vi "Main On Compile Action VI_Parse RTs.vi"(7 "Autocreate Rx timestamp chans?":bool, 8 "error in":errorcluster, 10 "Channel Ref":u64, 11 "Device Item Ref in":T3 format="%.0x") -> (0 "error out":errorcluster, 3 "RTs":T1[](array[typedef]) {"Mode Codes"."Words Item Refs" format="%.0x"; "Mode Codes"."Words Block Data Refs"."Data Reference" format="%.0x"; "Mode Codes"."Timestamp Channel Data Reference" format="%.0x"; "subAddresses"."Words Item Refs" format="%.0x"; "subAddresses"."Words Block Data Refs"."Data Reference" format="%.0x"; "subAddresses"."Timestamp Channel Data Reference" format="%.0x"; "Status Channel Data Reference" format="%.0x"; "Command Channels Refs" format="%.0x"})   [LabVIEW 2017, in "Ballard 1553 System Explorer.lvlib"]
uses:
  Ballard 1553 System Explorer.lvlib
  <vilib>/NI Veristand/Custom Device API/Custom Device Item Ref.ctl
  Shared/Controls and Global/RT Remote Terminal.ctl
  Shared/Controls and Global/RT Remote Terminal_rtMode.ctl
  <vilib>/NI Veristand/Custom Device API/Data Reference.ctl
  Shared/Controls and Global/RT Remote Terminal_RT subAddress.ctl
  Shared/Controls and Global/RT Remote Terminal_RT direction.ctl
  <vilib>/NI Veristand/Custom Device API/Block Data Reference.ctl
  Shared/Controls and Global/RT Remote Terminal_RT Mode Code.ctl
  Parse XML Ballard/Ballard_RT direction.ctl
  <vilib>/NI Veristand/Custom Device API/Data Access Type.ctl
  Shared/Controls and Global/Global.vi
  <vilib>/NI Veristand/Custom Device Tools/Custom Device Utility Library/NI VeriStand - Search for All Items by GUID.vi
  <vilib>/NI Veristand/Custom Device API/Get Item Property (I32).vi
  <vilib>/NI Veristand/Custom Device API/Get Item Property (U16).vi
  <vilib>/NI Veristand/Custom Device Tools/Custom Device Utility Library/NI VeriStand - Search for Item by Name.vi
  <vilib>/NI Veristand/Custom Device Tools/Custom Device Utility Library/NI VeriStand - Search for Item by GUID.vi
  Shared/Ballard 1553 Shared.lvlib
  <vilib>/NI VeriStand/Custom Device Tools/Custom Device Utility Library/Custom Device Utility Library.lvlib
  <vilib>/NI VeriStand/Custom Device API/Custom Device API.lvlib
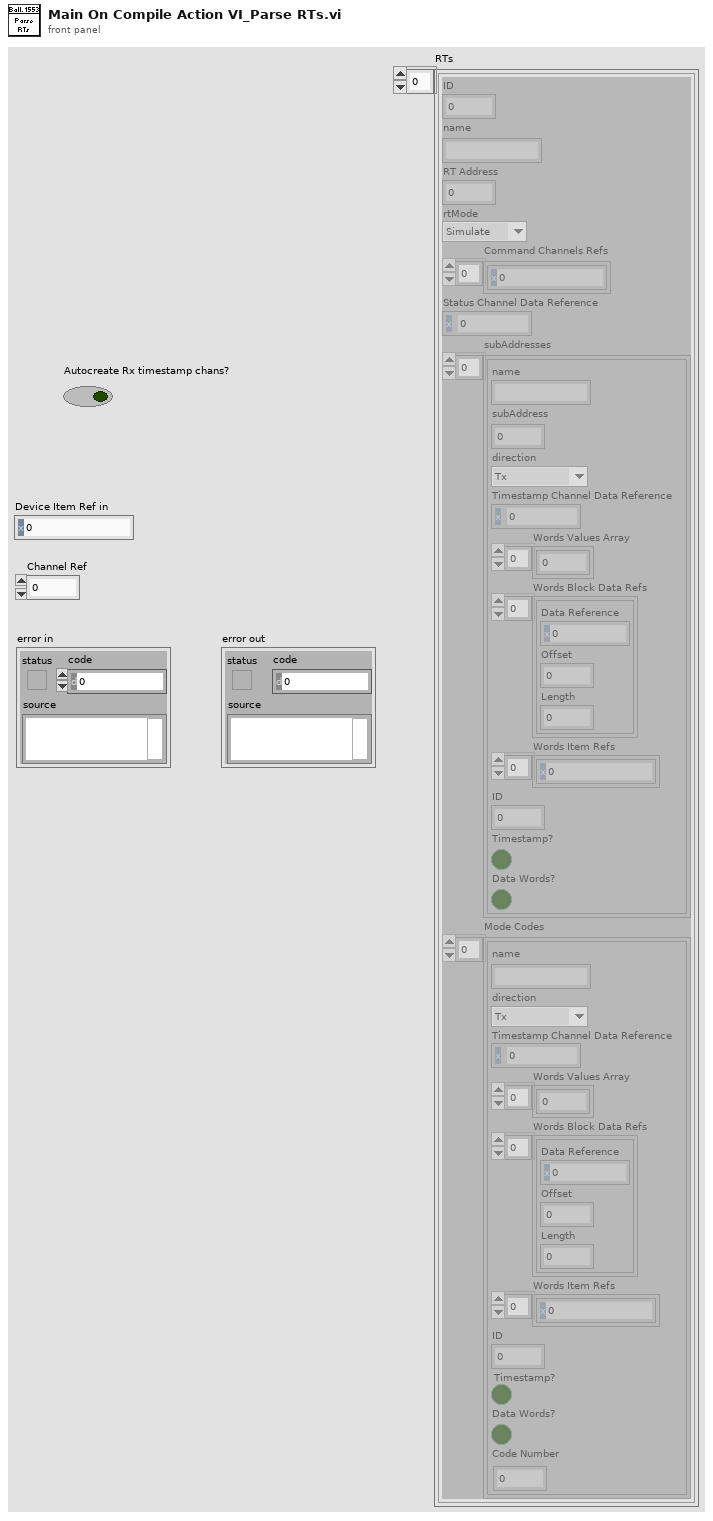
[diagram p1: front panel]
types:
  T1 = typedef "Ballard 1553 Shared.lvlib/RT Remote Terminal.ctl" = cluster{"ID":i32, "name":string, "RT Address":i32, "rtMode":T2, "Command Channels Refs":T3[], "Status Channel Data Reference":T4, "subAddresses":T5[], "Mode Codes":T8[]}
  T2 = typedef "Ballard 1553 Shared.lvlib/RT Remote Terminal_rtMode.ctl" = enum16{"Simulate", "Monitor", "Disable"}
  T3 = typedef "Custom Device API.lvlib/Custom Device Item Ref.ctl" = u64
  T4 = typedef "Custom Device API.lvlib/Data Reference.ctl" = i32
  T5 = typedef "Ballard 1553 Shared.lvlib/RT Remote Terminal_RT subAddress.ctl" = cluster{"name":string, "subAddress":i8, "direction":T6, "Timestamp Channel Data Reference":T4, "Words Values Array":u16[], "Words Block Data Refs":T7[], "Words Item Refs":T3[], "ID":i32, "Timestamp?":bool, "Data Words?":bool}
  T6 = typedef "Ballard 1553 Shared.lvlib/RT Remote Terminal_RT direction.ctl" = enum16{"Tx", "Rx"}
  T7 = typedef "Custom Device API.lvlib/Block Data Reference.ctl" = cluster{"Data Reference":T4, "Offset":u64, "Length":u64}
  T8 = typedef "Ballard 1553 Shared.lvlib/RT Remote Terminal_RT Mode Code.ctl" = cluster{"name":string, "direction":T6, "Timestamp Channel Data Reference":T4, "Words Values Array":u16[], "Words Block Data Refs":T7[], "Words Item Refs":T3[], "ID":i32, "Timestamp?":bool, "Data Words?":bool, "Code Number":i32}
  T9 = typedef "Custom Device API.lvlib/Data Access Type.ctl" = enum16{"Read", "Write"}
  T10 = typedef "Ballard 1553 System Explorer.lvlib/Ballard_RT direction.ctl" = enum16{"Tx", "Rx"}
  T11 = typedef "Custom Device API.lvlib/Custom Device Item Info.ctl" = cluster{"Name":string, "Is Channel":bool, "GUID":string, "Is Waveform":bool}
  T12 = typedef "Custom Device API.lvlib/Custom Device Channel.ctl" = cluster{"Type":T13, "Units":string, "Default Value":dbl, "Faultable":bool, "Scalable":bool}
  T13 = typedef "Custom Device API.lvlib/Custom Device Channel Type.ctl" = enum16{"Input", "Output"}
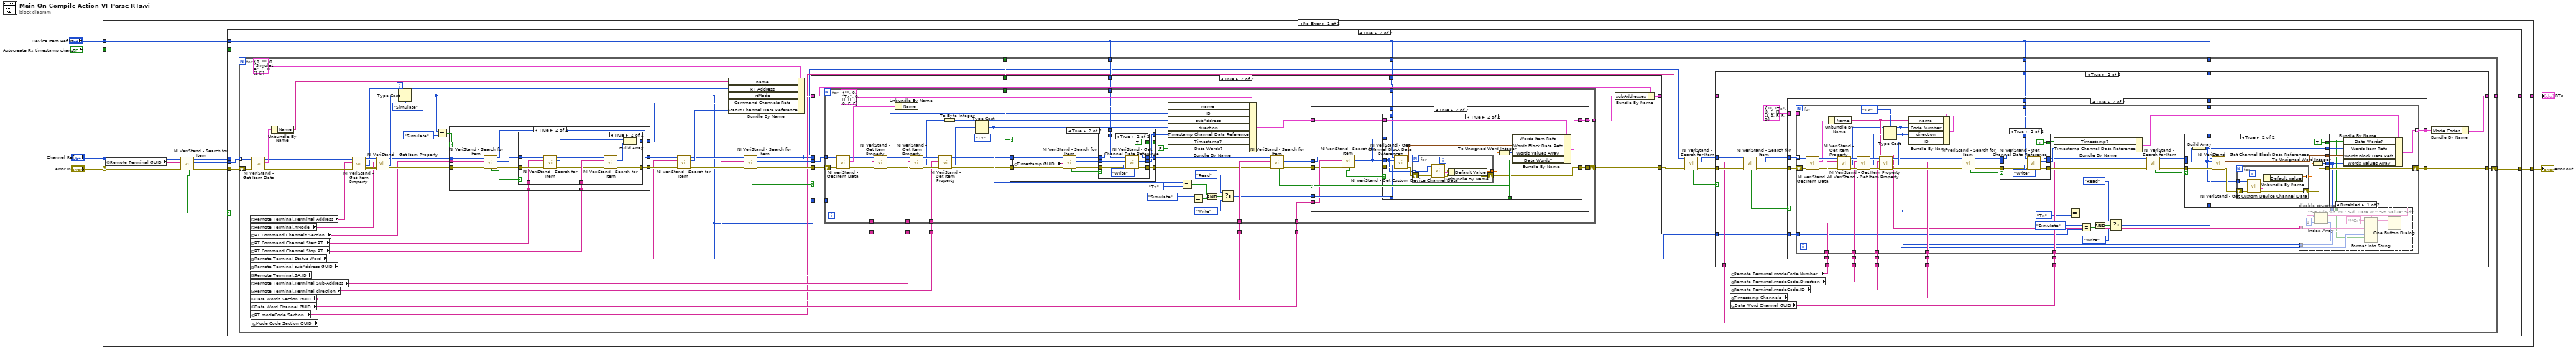
[diagram p0: block diagram]
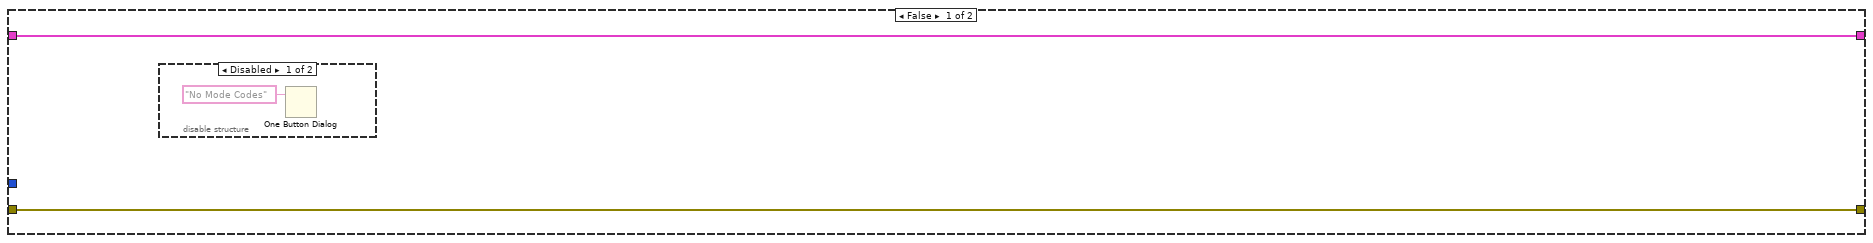
[diagram p3: hidden frame]
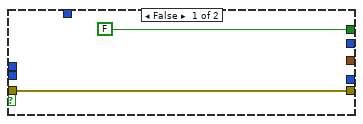
[diagram p7: hidden frame]
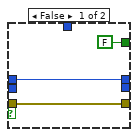
[diagram p8: hidden frame]
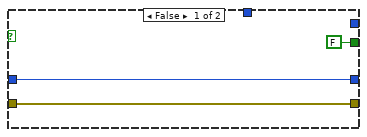
[diagram p12: hidden frame]
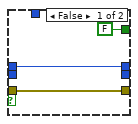
[diagram p13: hidden frame]
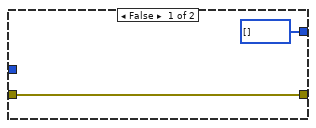
[diagram p15: hidden frame]
diagram:
  n1 = case shown="No Error" "error in" {
    selector: "error in" -> [w15 w362]
    tunnel: [w17 w362] -> w4
    tunnel: "Channel Ref" -> [w13 _]
    tunnel: "Autocreate Rx timestamp chans?" -> [w9 _]
    tunnel: "Device Item Ref in" -> [w8 _]
    tunnel: [w7 _] -> w1
    frame No Error {
      n2 = global read "Global.vi" "Remote Terminal GUID"() -> (w16:string)
      n3 = call-poly <vilib>:"NI VeriStand - Search for Item.vi"("error in"=w15, "Item GUID"=w16, "Section Ref in"=w13) -> ("error out"=w14:errorcluster, "Item Refs"=w10:T3[], "Section Ref out"=w12:T3, "Found"=w11:bool)  [unwired: 5 in]
      n4 = case shown="True" w11 {
        tunnel: [w18 w24] -> w17
        tunnel: w14 -> [w18 w23]
        tunnel: w12 -> [_ _]
        tunnel: w10 -> [_ w22]
        tunnel: w9 -> [_ w20]
        tunnel: w8 -> [_ w19]
        tunnel: [_ w21] -> w7
        frame False {
        }
        frame True {
          n5 = for {
            shift-right: [w35] -> w24
            shift-left: w23 -> [w83]
            tunnel: w22 -> [w82] mode=indexing
            tunnel: w19 -> [w49]
            tunnel: [w36] -> w21 mode=indexing
            tunnel: w20 -> [w48]
            tunnel: w19 -> [w46]
            tunnel: w19 -> [w28]
            tunnel: w19 -> [w26]
            n6 = global read "Global.vi" "Remote Terminal.Terminal Address"() -> (w73:string)
            n7 = global read "Global.vi" "Remote Terminal.rtMode"() -> (w74:string)
            n8 = global read "Global.vi" "RT.Command Channels Section"() -> (w68:string)
            n9 = global read "Global.vi" "RT.Command Channel.Start RT"() -> (w66:string)
            n10 = global read "Global.vi" "RT.Command Channel.Stop RT"() -> (w65:string)
            n11 = global read "Global.vi" "Remote Terminal Status Word"() -> (w60:string)
            n12 = global read "Global.vi" "Remote Terminal subAddress GUID"() -> (w55:string)
            n13 = global read "Global.vi" "Remote Terminal.SA.ID"() -> (w47:string)
            n14 = global read "Global.vi" "Remote Terminal.Terminal Sub-Address"() -> (w51:string)
            n15 = global read "Global.vi" "Remote Terminal.Terminal direction"() -> (w45:string)
            n16 = global read "Global.vi" "Data Words Section GUID"() -> (w44:string)
            n17 = global read "Global.vi" "Data Word Channel GUID"() -> (w43:string)
            n18 = global read "Global.vi" "RT.modeCode Section"() -> (w41:string)
            n19 = global read "Global.vi" "Mode Code Section GUID"() -> (w33:string)
            n20 = call <vilib>:"NI VeriStand - Get Item Data.vi"("error in (no error)"=w83, "Item Ref in"=w82) -> ("error out"=w77:errorcluster, "Item Info"=w81:T11, "Item Ref out"=w76:T3)  [unwired: 6 in, 1 out]
            n21 = Unbundle By Name(w81) -> ("Name"=w79:string)
            n22 = call-poly <vilib>:"NI VeriStand - Get Item Property.vi"("error in (no error)"=w77, "Property Name"=w73, "Item Ref in"=w76) -> ("error out"=w75:errorcluster, "Value"=w72:i32, "Item Ref out"=w78:T3)  [unwired: 5 in, 1 out]
            n23 = call-poly <vilib>:"NI VeriStand - Get Item Property.vi"("error in (no error)"=w75, "Property Name"=w74, "Item Ref in"=w78) -> ("error out"=w69:errorcluster, "Value"=w71:u16, "Item Ref out"=w67:T3)  [unwired: 5 in, 1 out]
            n24 = Type Cast(type=RT_Remote_Terminal_rtMode."Simulate" ("rtMode"), x=w71) -> (*(type *) &x=w25:T2)
            n25 = Equal?(x=w25, y=RT_Remote_Terminal_rtMode."Simulate" ("x")) -> (x = y?=w63:bool)
            n26 = case shown="True" w63 {
              tunnel: w69 -> [w338 w346]
              tunnel: w68 -> [_ w345]
              tunnel: w67 -> [w337 w344]
              tunnel: w66 -> [_ w343]
              tunnel: w65 -> [_ w342]
              tunnel: [_ w341] -> w64
              tunnel: [w338 w340] -> w61
              tunnel: [w337 w339] -> w59
              frame False {
                # "In Monitor Mode, these Channels don't exist."
              }
              frame True {
                n27 = call-poly <vilib>:"NI VeriStand - Search for Item.vi"("error in"=w346, "Item Name"=w345, "Section Ref in"=w344) -> ("error out"=w347:errorcluster, "Item Ref"=w349:T3, "Section Ref out"=w339:T3, "Found"=w348:bool)  [unwired: 5 in]
                n28 = case shown="True" w348 {
                  tunnel: w347 -> [w351 w361]
                  tunnel: w349 -> [_ w360]
                  tunnel: w343 -> [_ w359]
                  tunnel: w342 -> [_ w358]
                  tunnel: [w351 w355] -> w340
                  tunnel: [T3[] [] w352] -> w341
                  frame False {
                  }
                  frame True {
                    n29 = call-poly <vilib>:"NI VeriStand - Search for Item.vi"("error in"=w361, "Item Name"=w359, "Section Ref in"=w360) -> ("error out"=w356:errorcluster, "Item Ref"=w354:T3, "Section Ref out"=w357:T3)  [unwired: 5 in, 1 out]
                    n30 = call-poly <vilib>:"NI VeriStand - Search for Item.vi"("error in"=w356, "Item Name"=w358, "Section Ref in"=w357) -> ("error out"=w355:errorcluster, "Item Ref"=w353:T3)  [unwired: 5 in, 2 out]
                    n31 = Build Array(w354, w353) -> (w352:T3[])
                  }
                }
              }
            }
            n32 = call-poly <vilib>:"NI VeriStand - Search for Item.vi"("error in"=w61, "Item GUID"=w60, "Section Ref in"=w59) -> ("error out"=w56:errorcluster, "Item Ref"=w58:T3, "Section Ref out"=w57:T3)  [unwired: 5 in, 1 out]
            n33 = Bundle By Name(cluster=T1 {"ID"=0, "name"="", "RT Address"=0, "rtMode"=enum."Simulate", "Command Channels Refs"=[], "Status Channel Data Reference"=0, "subAddresses"=[], "Mode Codes"=[]} ("RT"), "name"=w79, "RT Address"=w72, "rtMode"=w25, "Command Channels Refs"=w64, "Status Channel Data Reference"=w58) -> (w50:T1)
            n34 = call-poly <vilib>:"NI VeriStand - Search for Item.vi"("error in"=w56, "Item GUID"=w55, "Section Ref in"=w57) -> ("error out"=w53:errorcluster, "Item Refs"=w52:T3[], "Section Ref out"=w40:T3, "Found"=w54:bool)  [unwired: 5 in]
            n35 = case shown="True" w54 {
              tunnel: w53 -> [w214 w228]
              tunnel: w52 -> [_ w229]
              tunnel: w40 -> [_ _]
              tunnel: [w214 w225] -> w42
              tunnel: w51 -> [_ w227]
              tunnel: w45 -> [_ w226]
              tunnel: w44 -> [_ w224]
              tunnel: w50 -> [w213 w223]
              tunnel: [w213 w221] -> w37
              tunnel: w25 -> [_ w220]
              tunnel: w49 -> [_ w219]
              tunnel: w48 -> [_ w218]
              tunnel: w47 -> [_ w217]
              tunnel: w46 -> [_ w216]
              tunnel: w43 -> [_ w215]
              frame False {
                # "No SAs found."
              }
              frame True {
                n36 = for {
                  tunnel: w229 -> [w274] mode=indexing
                  tunnel: w227 -> [w271]
                  tunnel: w226 -> [w270]
                  shift-right: [w257] -> w225
                  shift-left: w228 -> [w275]
                  tunnel: w224 -> [w263]
                  tunnel: [w258] -> w222 mode=indexing
                  tunnel: w220 -> [w245]
                  tunnel: w219 -> [w244]
                  tunnel: w218 -> [w241]
                  tunnel: w217 -> [w236]
                  tunnel: w216 -> [w233]
                  tunnel: w215 -> [w231]
                  n37 = call <vilib>:"NI VeriStand - Get Item Data.vi"("error in (no error)"=w275, "Item Ref in"=w274) -> ("error out"=w239:errorcluster, "Item Info"=w276:T11, "Item Ref out"=w240:T3)  [unwired: 6 in, 1 out]
                  n38 = call-poly <vilib>:"NI VeriStand - Get Item Property.vi"("error in (no error)"=w239, "Property Name"=w236, "Item Ref in"=w240) -> ("error out"=w237:errorcluster, "Value"=w234:i32, "Item Ref out"=w238:T3)  [unwired: 5 in, 1 out]
                  n39 = Unbundle By Name(w276) -> ("Name"=w235:string)
                  n40 = call-poly <vilib>:"NI VeriStand - Get Item Property.vi"("error in (no error)"=w237, "Property Name"=w271, "Item Ref in"=w238) -> ("error out"=w272:errorcluster, "Value"=w266:i32, "Item Ref out"=w273:T3)  [unwired: 5 in, 1 out]
                  n41 = call-poly <vilib>:"NI VeriStand - Get Item Property.vi"("error in (no error)"=w272, "Property Name"=w270, "Item Ref in"=w273) -> ("error out"=w255:errorcluster, "Value"=w268:u16, "Item Ref out"=w256:T3)  [unwired: 5 in, 1 out]
                  n42 = To Byte Integer(number=w266) -> (8bit integer=w265:i8)
                  n43 = Type Cast(type=RT_Remote_Terminal_RT_direction."Tx" ("direction"), x=w268) -> (*(type *) &x=w264:T6)
                  n44 = case shown="True" w241 {
                    tunnel: w256 -> [w312 w324]
                    tunnel: w255 -> [w313 w323]
                    tunnel: [_ w315] -> w254
                    tunnel: [w313 w318] -> w253
                    tunnel: [w312 w317] -> w252
                    tunnel: w233 -> [_ w316]
                    tunnel: [FALSE w314] -> w232
                    frame False {
                    }
                    frame True {
                      n45 = global read "Global.vi" "Timestamp GUID"() -> (w325:string)
                      n46 = call-poly <vilib>:"NI VeriStand - Search for Item.vi"("error in"=w323, "Item GUID"=w325, "Section Ref in"=w324) -> ("error out"=w321:errorcluster, "Item Ref"=w319:T3, "Section Ref out"=w320:T3, "Found"=w322:bool)  [unwired: 5 in]
                      n47 = case shown="True" w322 {
                        tunnel: w321 -> [w327 w333]
                        tunnel: w320 -> [w328 w336]
                        tunnel: w319 -> [_ w331]
                        tunnel: [w327 w332] -> w318
                        tunnel: [w328 w336] -> w317
                        tunnel: w316 -> [_ w334]
                        tunnel: [_ w330] -> w315
                        tunnel: [FALSE TRUE] -> w314
                        frame False {
                        }
                        frame True {
                          n48 = call <vilib>:"NI VeriStand - Get Channel Data Reference.vi"("error in (no error)"=w333, "Access"=Data_Access_Type."Write", "Channel Ref in"=w331, "Device Ref in"=w334) -> ("error out"=w332:errorcluster, "Channel Data Reference"=w330:T4)  [unwired: 5 in, 1 out]
                        }
                      }
                    }
                  }
                  n49 = Bundle By Name(cluster=T5 {"name"="", "subAddress"=0, "direction"=enum."Tx", "Timestamp Channel Data Reference"=0, "Words Values Array"=[], "Words Block Data Refs"=[], "Words Item Refs"=[], "ID"=0, "Timestamp?"=FALSE, "Data Words?"=FALSE} ("subAddress"), "name"=w235, "ID"=w234, "subAddress"=w265, "direction"=w264, "Timestamp Channel Data Reference"=w254, "Timestamp?"=w232, "Data Words?"=FALSE) -> (w260:T5)
                  n50 = Equal?(x=w264, y=Ballard_RT_direction."Tx") -> (x = y?=w249:bool)
                  n51 = Equal?(x=RT_Remote_Terminal_rtMode."Simulate", y=w245) -> (x = y?=w251:bool)
                  n52 = And(x=w249, y=w251) -> (x .and. y?=w248:bool)
                  n53 = Select(t=Data_Access_Type."Read" ("Access"), s=w248, f=Data_Access_Type."Write" ("Access")) -> (s? t:f=w246:T9)
                  n54 = call-poly <vilib>:"NI VeriStand - Search for Item.vi"("error in"=w253, "Item GUID"=w263, "Section Ref in"=w252) -> ("error out"=w261:errorcluster, "Item Ref"=w259:T3, "Found"=w262:bool)  [unwired: 5 in, 1 out]
                  n55 = case shown="True" w262 {
                    selector: w262 -> [_ w285]
                    tunnel: w261 -> [w277 w282]
                    tunnel: w260 -> [w278 w290]
                    tunnel: [w278 w289] -> w258
                    tunnel: w259 -> [_ w284]
                    tunnel: [w277 w288] -> w257
                    tunnel: w246 -> [_ w286]
                    tunnel: w244 -> [_ w287]
                    tunnel: w231 -> [_ w283]
                    frame False {
                    }
                    frame True {
                      n56 = call-poly <vilib>:"NI VeriStand - Search for Item.vi"("error in"=w282, "Item GUID"=w283, "Section Ref in"=w284) -> ("error out"=w280:errorcluster, "Item Refs"=w279:T3[], "Found"=w281:bool)  [unwired: 5 in, 1 out]
                      n57 = case shown="True" w281 {
                        tunnel: w290 -> [w292 w305]
                        tunnel: [w292 w304] -> w289
                        tunnel: [w291 w295] -> w288
                        tunnel: w287 -> [_ w302]
                        tunnel: w286 -> [_ w301]
                        tunnel: w285 -> [_ w299]
                        tunnel: w280 -> [w291 w298]
                        tunnel: w279 -> [_ w293]
                        tunnel: w279 -> [_ w297]
                        frame False {
                        }
                        frame True {
                          n58 = call <vilib>:"NI VeriStand - Get Channel Block Data References.vi"("error in (no error)"=w298, "Access"=w301, "Channel Refs"=w293, "Device Ref in"=w302) -> ("error out"=w296:errorcluster, "Block Data Refs"=w303:T7[])  [unwired: 4 in, 2 out]
                          n59 = for {
                            tunnel: [w306] -> w294 mode=indexing
                            shift-right: [w307] -> w295
                            shift-left: w296 -> [w310]
                            tunnel: w293 -> [w308] mode=indexing
                            n60 = call <vilib>:"NI VeriStand - Get Custom Device Channel Data.vi"("error in (no error)"=w310, "Channel Ref in"=w308) -> ("error out"=w307:errorcluster, "Channel"=w309:T12)  [unwired: 4 in, 4 out]
                            n61 = Unbundle By Name(w309) -> ("Default Value"=w306:dbl)
                          }
                          n62 = To Unsigned Word Integer(number=w294) -> (unsigned 16bit integer=w300:u16[])
                          n63 = Bundle By Name(cluster=w305, "Words Item Refs"=w297, "Words Block Data Refs"=w303, "Words Values Array"=w300, "Data Words?"=w299) -> (w304:T5)
                        }
                      }
                    }
                  }
                }
                n64 = Bundle By Name(cluster=w223, "subAddresses"=w222) -> (w221:T1)
              }
            }
            n65 = call-poly <vilib>:"NI VeriStand - Search for Item.vi"("error in"=w42, "Item Name"=w41, "Section Ref in"=w40) -> ("error out"=w39:errorcluster, "Item Ref"=w34:T3, "Found"=w38:bool)  [unwired: 5 in, 1 out]
            n66 = global read "Global.vi" "Remote Terminal.modeCode.Number"() -> (w32:string)
            n67 = global read "Global.vi" "Remote Terminal.modeCode.Direction"() -> (w31:string)
            n68 = global read "Global.vi" "Remote Terminal.modeCode.ID"() -> (w30:string)
            n69 = global read "Global.vi" "Timestamp Channels"() -> (w29:string)
            n70 = global read "Global.vi" "Data Word Channel GUID"() -> (w27:string)
            n71 = case shown="True" w38 {
              tunnel: w39 -> [w84 w105]
              tunnel: w37 -> [w85 w99]
              tunnel: [w85 w98] -> w36
              tunnel: [w84 w100] -> w35
              tunnel: w34 -> [_ w103]
              tunnel: w33 -> [_ w104]
              tunnel: w32 -> [_ w96]
              tunnel: w31 -> [_ w95]
              tunnel: w30 -> [_ w94]
              tunnel: w29 -> [_ w93]
              tunnel: w28 -> [_ w92]
              tunnel: w27 -> [_ w90]
              tunnel: w26 -> [_ w89]
              tunnel: w25 -> [_ w88]
              frame False {
                n72 = disable-structure shown="Disabled" {
                  frame Disabled {
                    n73 = One Button Dialog(message="No Mode Codes") -> ()  [unwired: 1 in, 1 out]
                  }
                  frame Enabled {
                  }
                }
              }
              frame True {
                n74 = call-poly <vilib>:"NI VeriStand - Search for Item.vi"("error in"=w105, "Item GUID"=w104, "Section Ref in"=w103) -> ("error out"=w101:errorcluster, "Item Refs"=w87:T3[], "Found"=w102:bool)  [unwired: 5 in, 1 out]
                n75 = case shown="True" w102 {
                  tunnel: w87 -> [_ w119]
                  tunnel: w101 -> [w106 w118]
                  tunnel: [w106 w117] -> w100
                  tunnel: T8 {"name"="", "direction"=enum."Tx", "Timestamp Channel Data Reference"=0, "Words Values Array"=[], "Words Block Data Refs"=[], "Words Item Refs"=[], "ID"=0, "Timestamp?"=FALSE, "Data Words?"=FALSE, "Code Number"=0} ("subAddress") -> [_ w116]
                  tunnel: w96 -> [_ w115]
                  tunnel: w95 -> [_ w114]
                  tunnel: w94 -> [_ w113]
                  tunnel: w93 -> [_ w112]
                  tunnel: w92 -> [_ w111]
                  tunnel: [_ w110] -> w91
                  tunnel: w90 -> [_ w109]
                  tunnel: w89 -> [_ w108]
                  tunnel: w88 -> [_ w107]
                  frame False {
                  }
                  frame True {
                    n76 = for {
                      tunnel: w119 -> [w169] mode=indexing
                      shift-right: [w144] -> w117
                      shift-left: w118 -> [w163]
                      tunnel: w116 -> [w165]
                      tunnel: w115 -> [w168]
                      tunnel: w114 -> [w167]
                      tunnel: w113 -> [w166]
                      tunnel: w112 -> [w155]
                      tunnel: w111 -> [w150]
                      tunnel: [w142] -> w110 mode=indexing
                      tunnel: w109 -> [w141]
                      tunnel: w108 -> [w139]
                      tunnel: w107 -> [w129]
                      n77 = call <vilib>:"NI VeriStand - Get Item Data.vi"("error in (no error)"=w163, "Item Ref in"=w169) -> ("error out"=w162:errorcluster, "Item Info"=w161:T11, "Item Ref out"=w164:T3)  [unwired: 6 in, 1 out]
                      n78 = Unbundle By Name(w161) -> ("Name"=w124:string)
                      n79 = call-poly <vilib>:"NI VeriStand - Get Item Property.vi"("error in (no error)"=w162, "Property Name"=w168, "Item Ref in"=w164) -> ("error out"=w173:errorcluster, "Value"=w122:i32, "Item Ref out"=w172:T3)  [unwired: 5 in, 1 out]
                      n80 = call-poly <vilib>:"NI VeriStand - Get Item Property.vi"("error in (no error)"=w173, "Property Name"=w167, "Item Ref in"=w172) -> ("error out"=w171:errorcluster, "Value"=w159:u16, "Item Ref out"=w170:T3)  [unwired: 5 in, 1 out]
                      n81 = call-poly <vilib>:"NI VeriStand - Get Item Property.vi"("error in (no error)"=w171, "Property Name"=w166, "Item Ref in"=w170) -> ("error out"=w157:errorcluster, "Value"=w158:i32, "Item Ref out"=w156:T3)  [unwired: 5 in, 1 out]
                      n82 = Type Cast(type=RT_Remote_Terminal_RT_direction."Tx" ("direction"), x=w159) -> (*(type *) &x=w123:T6)
                      n83 = Bundle By Name(cluster=w165, "name"=w124, "Code Number"=w122, "direction"=w123, "ID"=w158) -> (w154:T8)
                      n84 = call-poly <vilib>:"NI VeriStand - Search for Item.vi"("error in"=w157, "Item Name"=w155, "Section Ref in"=w156) -> ("error out"=w153:errorcluster, "Item Ref"=w151:T3, "Section Ref out"=w152:T3, "Found"=w127:bool)  [unwired: 5 in]
                      n85 = case shown="True" w127 {
                        tunnel: w153 -> [w204 w210]
                        tunnel: w152 -> [w202 w212]
                        tunnel: [w204 w209] -> w145
                        tunnel: [w202 w212] -> w140
                        tunnel: [_ w208] -> w149
                        tunnel: [FALSE TRUE] -> w126
                        tunnel: w151 -> [_ w206]
                        tunnel: w150 -> [_ w205]
                        frame False {
                        }
                        frame True {
                          n86 = call <vilib>:"NI VeriStand - Get Channel Data Reference.vi"("error in (no error)"=w210, "Access"=Data_Access_Type."Write", "Channel Ref in"=w206, "Device Ref in"=w205) -> ("error out"=w209:errorcluster, "Channel Data Reference"=w208:T4)  [unwired: 5 in, 1 out]
                        }
                      }
                      n87 = Bundle By Name(cluster=w154, "Timestamp?"=w126, "Timestamp Channel Data Reference"=w149) -> (w143:T8)
                      n88 = Equal?(x=w123, y=Ballard_RT_direction."Tx") -> (x = y?=w134:bool)
                      n89 = Equal?(x=RT_Remote_Terminal_rtMode."Simulate", y=w129) -> (x = y?=w136:bool)
                      n90 = And(x=w134, y=w136) -> (x .and. y?=w133:bool)
                      n91 = Select(t=Data_Access_Type."Read" ("Access"), s=w133, f=Data_Access_Type."Write" ("Access")) -> (s? t:f=w130:T9)
                      n92 = call-poly <vilib>:"NI VeriStand - Search for Item.vi"("error in"=w145, "Item GUID"=w141, "Section Ref in"=w140) -> ("error out"=w146:errorcluster, "Item Ref"=w148:T3, "Section Ref out"=w147:T3, "Found"=w125:bool)  [unwired: 5 in]
                      n93 = case shown="True" w125 {
                        tunnel: w146 -> [w185 w196]
                        tunnel: w147 -> [_ _]
                        tunnel: [w185 w187] -> w144
                        tunnel: [FALSE TRUE] -> w121
                        tunnel: w148 -> [_ w193]
                        tunnel: w139 -> [_ w194]
                        tunnel: [_ w188] -> w138
                        tunnel: [_ w192] -> w120
                        tunnel: [_ w191] -> w137
                        tunnel: w130 -> [_ w190]
                        frame False {
                        }
                        frame True {
                          n94 = Build Array(w193) -> (w188:T3[])
                          n95 = call <vilib>:"NI VeriStand - Get Channel Block Data References.vi"("error in (no error)"=w196, "Access"=w190, "Channel Refs"=w188, "Device Ref in"=w194) -> ("error out"=w189:errorcluster, "Block Data Refs"=w191:T7[])  [unwired: 4 in, 2 out]
                          n96 = for {
                            tunnel: [w197] -> w186 mode=indexing
                            shift-right: [w198] -> w187
                            shift-left: w189 -> [w201]
                            tunnel: w188 -> [w199] mode=indexing
                            n97 = call <vilib>:"NI VeriStand - Get Custom Device Channel Data.vi"("error in (no error)"=w201, "Channel Ref in"=w199) -> ("error out"=w198:errorcluster, "Channel"=w200:T12)  [unwired: 4 in, 4 out]
                            n98 = Unbundle By Name(w200) -> ("Default Value"=w197:dbl)
                          }
                          n99 = To Unsigned Word Integer(number=w186) -> (unsigned 16bit integer=w192:u16[])
                        }
                      }
                      n100 = disable-structure shown="Disabled" {
                        disable-tunnel: w124 -> [w181 _]
                        disable-tunnel: w123 -> [w180 _]
                        disable-tunnel: w122 -> [w179 _]
                        disable-tunnel: w121 -> [w178 _]
                        disable-tunnel: w120 -> [w177 _]
                        frame Disabled {
                          n101 = Index Array(array=w177, index=0) -> (element=w175:u16)
                          n102 = Format Into String(format string="%s, Dir: %s, MC: %d, Data W?: %s, Value: %d", initial string="MC: ", w181, w180, w179, w178, w175) -> (resulting string=w183:string)  [unwired: 1 in, 1 out]
                          n103 = One Button Dialog(message=w183) -> ()  [unwired: 1 in, 1 out]
                        }
                        frame Enabled {
                        }
                      }
                      n104 = Bundle By Name(cluster=w143, "Data Words?"=w121, "Words Item Refs"=w138, "Words Block Data Refs"=w137, "Words Values Array"=w120) -> (w142:T8)
                    }
                  }
                }
                n105 = Bundle By Name(cluster=w99, "Mode Codes"=w91) -> (w98:T1)
              }
            }
          }
        }
      }
    }
    frame Error {
    }
  }
  "error out" <- w4
  "RTs" <- w1
